vi "generate full alarm table.vi"(7 "Full Alarms Table":refnum<vi>, 8 "error in":errorcluster, 10 "engine configuration":refnum<class "engine configuration.lvclass">, 11 "tag bus configurable plugin module configuration":refnum<class "alarms module configuration.lvclass">) -> (0 "error out":errorcluster)   [LabVIEW 2013, in "alarms module editor node.lvclass"]
uses:
  alarms module editor node.lvclass
  module/configuration/alarms module configuration.lvclass
  <vilib>/NI/Module Execution Interface/Engine Configuration/engine configuration.lvclass
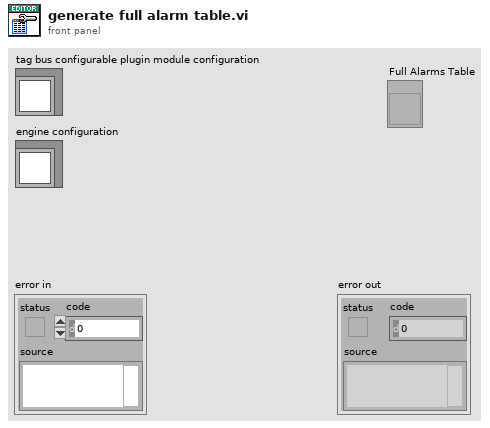
[diagram p1: front panel]
types:
  T1 = typedef "alarms module configuration.lvclass/alarm configuration.ctl" = cluster{"alarm name":string, "comparisons":T2[], "unlatch":refnum<class "TBM channel.lvclass">, "output":refnum<class "TBM channel.lvclass">, "boolean op":T4}
  T2 = typedef "alarms module configuration.lvclass/alarm comparison.ctl" = cluster{"input channel":refnum<class "TBM channel.lvclass">, "limit":dbl, "comparison":T3}
  T3 = typedef "alarms module configuration.lvclass/compare type.ctl" = enum16{">", "<", ">=", "<=", "="}
  T4 = typedef "alarms module configuration.lvclass/boolean operation.ctl" = enum16{"AND", "OR"}
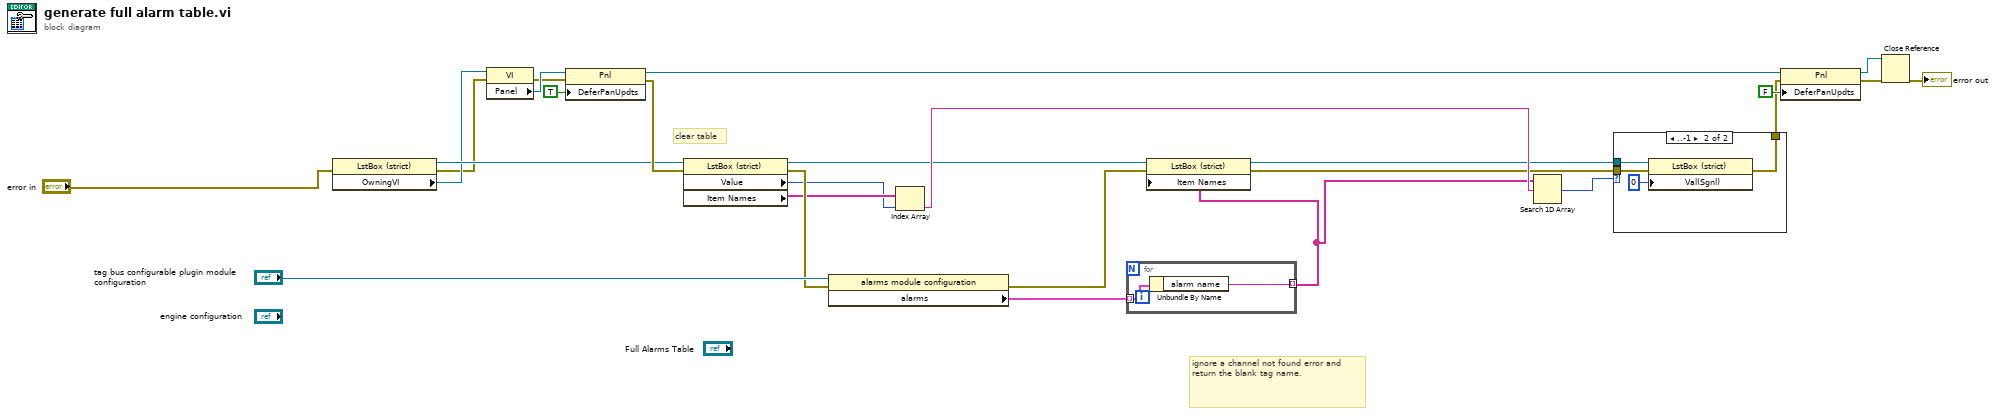
[diagram p0: block diagram]
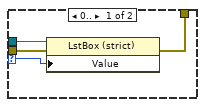
[diagram p2: hidden frame]
diagram:
  # "ignore a channel not found error and return the blank tag name."
  # "clear table"
  n1 = property class="LstBox (strict)"(error in="error in") -> (reference=w10:refnum<vi>, reference out=w16:refnum<vi>, error out=w13:errorcluster, "OwningVI"=w14:refnum<vi>)
  n2 = property class="VI"(reference=w14, error in=w13) -> (error out=w22:errorcluster, "Panel"=w23:refnum<vi>)  [unwired: 1 out]
  n3 = property class="Pnl"(reference=w23, error in=w22, "DeferPanUpdts"=TRUE ("Defer Panel Updates")) -> (reference out=w19:refnum<vi>, error out=w21:errorcluster)
  n4 = property class="LstBox (strict)"(reference=w16, error in=w21) -> (reference out=w5:refnum<vi>, error out=w25:errorcluster, "Value"=w8:i32, "Item Names"=w9:string[])
  n5 = property class="alarms module configuration"(reference="tag bus configurable plugin module configuration", error in=w25) -> (error out=w3:errorcluster, "alarms"=w26:T1[])  [unwired: 1 out]
  n6 = Index Array(array=w9, index=w8) -> (element=w6:string)
  n7 = for {
    tunnel: w26 -> [w29] mode=indexing
    tunnel: [w28] -> w1 mode=indexing
    n8 = Unbundle By Name(w29) -> ("alarm name"=w28:string)
  }
  n9 = property class="LstBox (strict)"(reference=w5, error in=w3, "Item Names"=w1) -> (reference out=w4:refnum<vi>, error out=w2:errorcluster)
  n10 = Search 1D Array(1D array=w1, element=w6) -> (index of element=w7:i32)  [unwired: 1 in]
  n11 = case shown="..-1" w7 {
    selector: w7 -> [w30 _]
    tunnel: w4 -> [w33 w37]
    tunnel: w2 -> [w32 w36]
    tunnel: [w31 w35] -> w18
    frame 0.. {
      n12 = property class="LstBox (strict)"(reference=w33, error in=w32, "Value"=w30) -> (error out=w31:errorcluster)  [unwired: 1 out]
    }
    frame ..-1 {
      n13 = property class="LstBox (strict)"(reference=w37, error in=w36, "Val(Sgnl)"=0 ("Value (Signaling)")) -> (error out=w35:errorcluster)  [unwired: 1 out]
    }
  }
  n14 = property class="Pnl"(reference=w19, error in=w18, "DeferPanUpdts"=FALSE ("Defer Panel Updates")) -> (reference out=w11:refnum<vi>, error out=w17:errorcluster)
  n15 = Close Reference(reference=w11, error in (no error)=w17) -> (error out=→"error out":errorcluster)
